vi "ResetTeserBeforePowerON (SubVI).vi"(8 "error in (no error)":errorcluster, 11 "DAQmx Device Name":tag) -> (0 "error out":errorcluster)   [LabVIEW 2017]
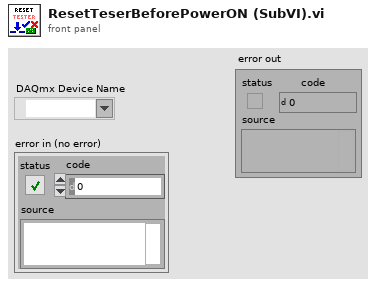
[diagram p1: front panel]
types:
  T1 = enum16{"DB0", "DB1", "DB2", "DB3", "DB4", "DB5", "DB6", "DB7", "DB8", "DB9", "DB10", "DB11", "A0", "A1", "RW", "LDAC", "ADMAIN1", "ADMAIN2", "ADMAIN3", "G1", "CS", "CLR", "P0", "P1"}
  T2 = enum16{"Reset", "Update U1", "Update U2", "Update U3", "Read all"}
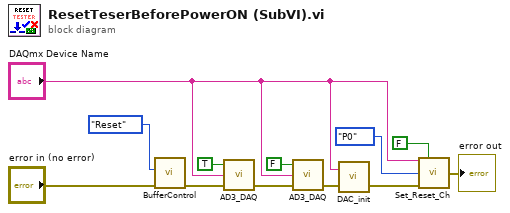
[diagram p0: block diagram]
diagram:
  n1 = call "BufferControl.vi"("error in"="error in (no error)", "Enum"=T2."Reset") -> ("error out"=w5:errorcluster)  [unwired: 2 in, 3 out]
  n2 = call "AD3_DAQ.vi"("error in"=w5, "device name"="DAQmx Device Name", "Boolean In"=TRUE) -> ("error out"=w4:errorcluster)  [unwired: 2 in]
  n3 = call "AD3_DAQ.vi"("error in"=w4, "device name"="DAQmx Device Name", "Boolean In"=FALSE) -> ("error out"=w3:errorcluster)  [unwired: 2 in]
  n4 = call "DAC_init.vi"("error in"=w3, "device name"="DAQmx Device Name") -> ("error out"=w2:errorcluster)  [unwired: 1 in]
  n5 = call "Set_Reset_Ch.vi"("device name"="DAQmx Device Name", "SetReset"=FALSE, "Ch"=T1."P0" ("Ch 2"), "error in"=w2) -> ("error out"=→"error out":errorcluster)  [unwired: 11 in]
